vi "classify error.vi"(8 "error to classify":errorcluster, 11 "Scan Engine runtime in":refnum<class "Scan Engine runtime.lvclass">) -> (0 "classified error":errorcluster, 2 "error classification":T1, 3 "Scan Engine runtime out":refnum<class "Scan Engine runtime.lvclass">)   [LabVIEW 2013, in "Scan Engine runtime.lvclass"]
doc: "Allows a module to classify an error generated at any point during execution. This <b>error classification</b> can then be used by calling code to determine if execution can continue. In addition, this function can be used to allow a component to clear an error, convert an error to a warning, or attempt to recover from an error. Recovery may be attempted only if <b>attempt recovery?</b> is true."
uses:
  Scan Engine runtime.lvclass
  <vilib>/NI/Tag Bus Module Framework/runtime/error classification.ctl
  <vilib>/NI/Tag Bus Module Framework/runtime/TBM module execution interface.lvclass
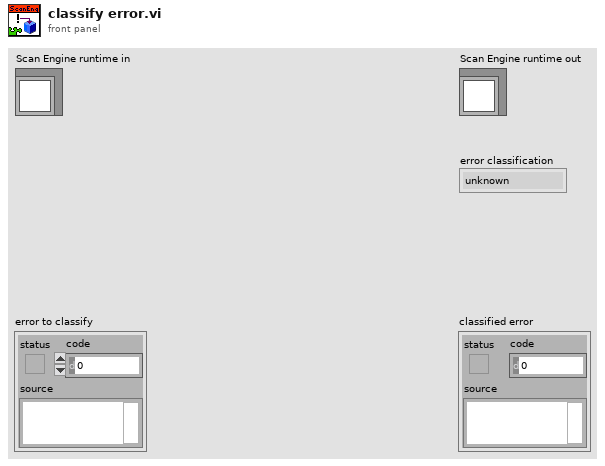
[diagram p1: front panel]
types:
  T1 = typedef "TBM module execution interface.lvclass/error classification.ctl" = enum16{"unknown", "none", "trivial", "recoverable", "critical"}
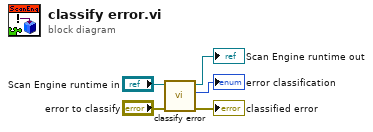
[diagram p0: block diagram]
diagram:
  n1 = call-parent "classify error.vi"("error to classify"="error to classify", "module in"="Scan Engine runtime in") -> ("classified error"=→"classified error":errorcluster, "error classification"=→"error classification":T1, "module out"=→"Scan Engine runtime out":refnum<class "Scan Engine runtime.lvclass">)  [unwired: 7 in]
